vi "AI Read Body.vi"(6 "error in":errorcluster, 9 "Channel":tag) -> (0 "error out":errorcluster, 2 "data":dbl format="%0.2f")   [LabVIEW 2015, in "DAQ.lvlib"]
uses:
  DAQ.lvlib
  <vilib>/DAQmx/create/channels.llb/DAQmx Create Channel (AI-Voltage-Basic).vi
  <vilib>/DAQmx/read.llb/DAQmx Read (Analog DBL 1Chan 1Samp).vi
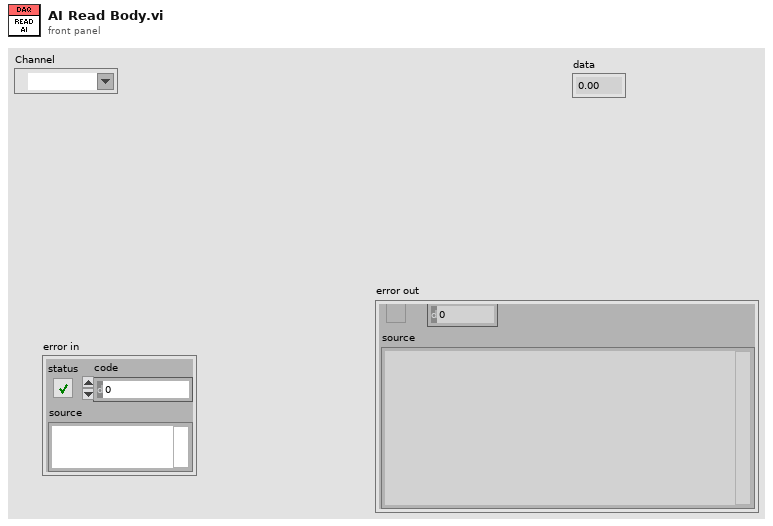
[diagram p1: front panel]
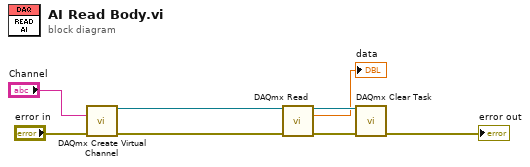
[diagram p0: block diagram]
diagram:
  n1 = call-poly <vilib>:"DAQmx Create Virtual Channel.vi"("physical channels"="Channel", "error in"="error in") -> ("task out"=w8:refnum<k21>, "error out"=w7:errorcluster)  [unwired: 12 in]
  n2 = call-poly <vilib>:"DAQmx Read.vi"("task/channels in"=w8, "error in"=w7) -> ("task out"=w6:refnum<k21>, "data"=→"data":dbl, "error out"=w5:errorcluster)  [unwired: 11 in]
  n3 = call <vilib>:"DAQmx Clear Task.vi"("task in"=w6, "error in"=w5) -> ("error out"=→"error out":errorcluster)  [unwired: 13 in]
